vi "HandleSuffix.vi"(8 "error in (no error)":errorcluster, 11 "S4GUI in":refnum<class "S4GUI.lvclass">) -> (0 "error out":errorcluster, 3 "S4GUI out":refnum<class "S4GUI.lvclass">)   [LabVIEW 2018, in "S4GUI.lvclass"]
uses:
  S4GUI.lvclass
  S4GUI.lvclass/S4GUI.ctl
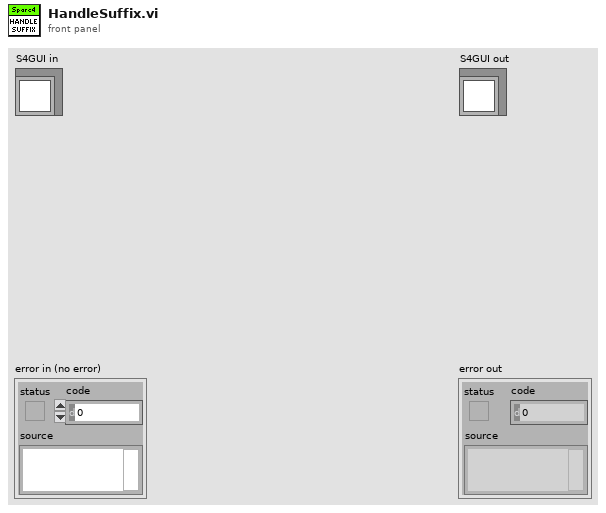
[diagram p1: front panel]
types:
  T1 = enum32{"OBJECT", "TEST", "DFLAT", "SFLAT", "DARK", "ZERO", "FOCUS"}
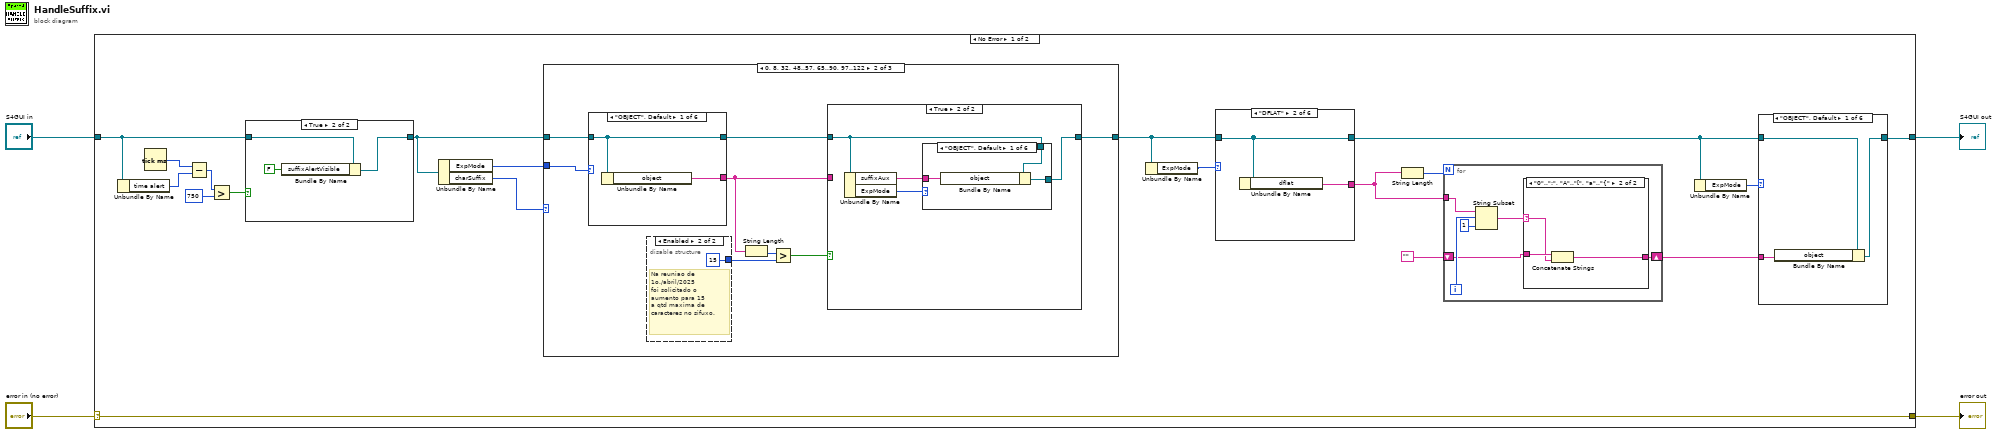
[diagram p0: block diagram]
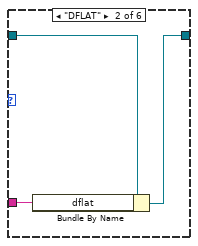
[diagram p2: hidden frame]
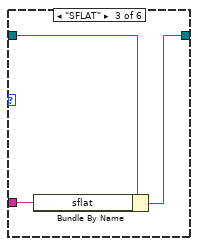
[diagram p3: hidden frame]
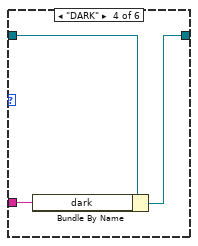
[diagram p4: hidden frame]
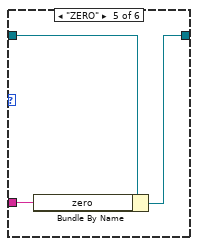
[diagram p5: hidden frame]
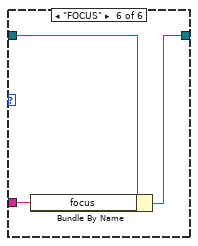
[diagram p6: hidden frame]
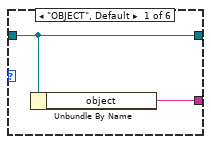
[diagram p8: hidden frame]
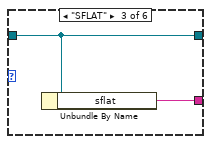
[diagram p9: hidden frame]
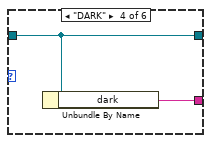
[diagram p10: hidden frame]
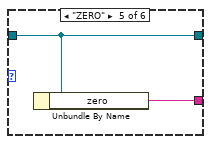
[diagram p11: hidden frame]
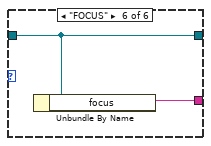
[diagram p12: hidden frame]
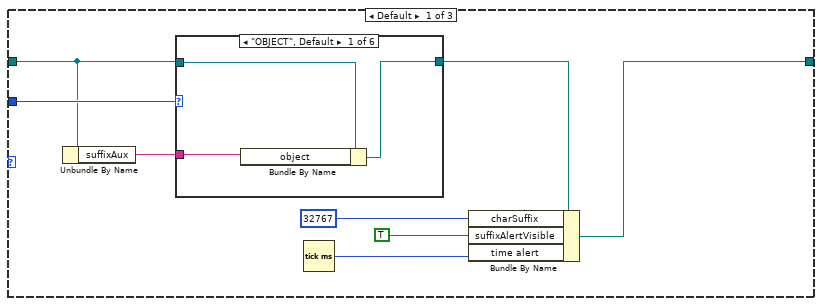
[diagram p13: hidden frame]
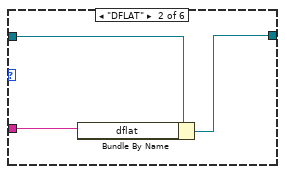
[diagram p14: hidden frame]
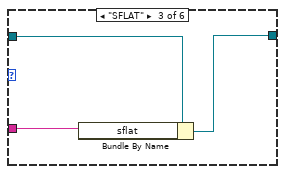
[diagram p15: hidden frame]
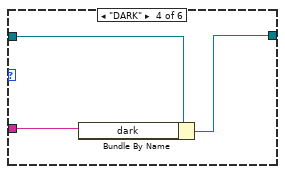
[diagram p16: hidden frame]
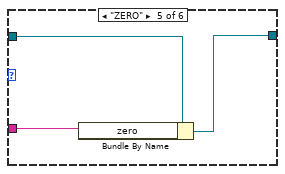
[diagram p17: hidden frame]
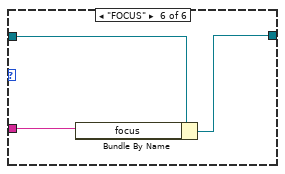
[diagram p18: hidden frame]
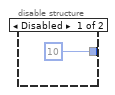
[diagram p19: hidden frame]
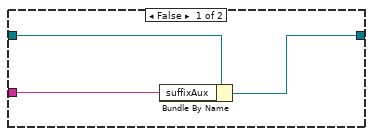
[diagram p20: hidden frame]
diagram:
  n1 = case shown="No Error" "error in (no error)" {
    selector: "error in (no error)" -> [w23 w143]
    tunnel: [w23 w143] -> w3
    tunnel: [w6 w142] -> w1
    tunnel: "S4GUI in" -> [w18 w142]
    frame No Error {
      n2 = Unbundle By Name(w18) -> ("time alert"=w20:u32)
      n3 = Tick Count (ms)() -> (millisecond timer value=w21:u32)
      n4 = Subtract(x=w21, y=w20) -> (x-y=w22:u32)
      n5 = Greater?(x=w22, y=u32 750) -> (0:w17:bool)
      n6 = case shown="True" w17 {
        tunnel: w18 -> [w138 w141]
        tunnel: [w138 w140] -> w15
        frame False {
        }
        frame True {
          n7 = Bundle By Name(cluster=w141, "suffixAlertVisible"=FALSE) -> (w140:refnum<class "S4GUI.lvclass">)
        }
      }
      n8 = Unbundle By Name(w15) -> ("ExpMode"=w16:T1, "charSuffix"=w14:i16)
      n9 = case shown="0, 8, 32, 48..57, 65..90, 97..122" w14 {
        tunnel: w15 -> [w70 w97 w137]
        tunnel: w16 -> [w71 w96 _]
        tunnel: [w64 w91 w137] -> w12
        frame Default {
          n10 = Unbundle By Name(w70) -> ("suffixAux"=w69:string)
          n11 = case shown="\"OBJECT\", Default" w71 {
            tunnel: w70 -> [w74 w77 w80 w83 w86 w89]
            tunnel: [w73 w76 w79 w82 w85 w88] -> w68
            tunnel: w69 -> [w72 w75 w78 w81 w84 w87]
            frame "OBJECT", Default {
              n12 = Bundle By Name(cluster=w74, "object"=w72) -> (w73:refnum<class "S4GUI.lvclass">)
            }
            frame "DFLAT" {
              n13 = Bundle By Name(cluster=w77, "dflat"=w75) -> (w76:refnum<class "S4GUI.lvclass">)
            }
            frame "SFLAT" {
              n14 = Bundle By Name(cluster=w80, "sflat"=w78) -> (w79:refnum<class "S4GUI.lvclass">)
            }
            frame "DARK" {
              n15 = Bundle By Name(cluster=w83, "dark"=w81) -> (w82:refnum<class "S4GUI.lvclass">)
            }
            frame "ZERO" {
              n16 = Bundle By Name(cluster=w86, "zero"=w84) -> (w85:refnum<class "S4GUI.lvclass">)
            }
            frame "FOCUS" {
              n17 = Bundle By Name(cluster=w89, "focus"=w87) -> (w88:refnum<class "S4GUI.lvclass">)
            }
          }
          n18 = Tick Count (ms)() -> (millisecond timer value=w65:u32)
          n19 = Bundle By Name(cluster=w68, "charSuffix"=i16 32767, "suffixAlertVisible"=TRUE, "time alert"=w65) -> (w64:refnum<class "S4GUI.lvclass">)
        }
        frame 0, 8, 32, 48..57, 65..90, 97..122 {
          n20 = case shown="\"OBJECT\", Default" w96 {
            tunnel: w97 -> [w126 w128 w130 w132 w134 w136]
            tunnel: [w126 w128 w130 w132 w134 w136] -> w92
            tunnel: [w125 w127 w129 w131 w133 w135] -> w90
            frame "OBJECT", Default {
              n21 = Unbundle By Name(w126) -> ("object"=w125:string)
            }
            frame "DFLAT" {
              n22 = Unbundle By Name(w128) -> ("dflat"=w127:string)
            }
            frame "SFLAT" {
              n23 = Unbundle By Name(w130) -> ("sflat"=w129:string)
            }
            frame "DARK" {
              n24 = Unbundle By Name(w132) -> ("dark"=w131:string)
            }
            frame "ZERO" {
              n25 = Unbundle By Name(w134) -> ("zero"=w133:string)
            }
            frame "FOCUS" {
              n26 = Unbundle By Name(w136) -> ("focus"=w135:string)
            }
          }
          n27 = disable-structure shown="Enabled" {
            disable-tunnel: [10 ("y") 15 ("y")] -> w94
            frame Disabled {
            }
            frame Enabled {
              # "Na reuniao de \n1o./abril/2025\nfoi solicitado o \naumento para 15\na qtd maxima de\ncaracteres no sifuxo."
            }
          }
          n28 = String Length(string=w90) -> (length=w95:i32)
          n29 = Greater?(x=w95, y=w94) -> (0:w93:bool)
          n30 = case shown="True" w93 {
            tunnel: w92 -> [w102 w106]
            tunnel: [w101 w105] -> w91
            tunnel: w90 -> [w100 _]
            frame False {
              n31 = Bundle By Name(cluster=w102, "suffixAux"=w100) -> (w101:refnum<class "S4GUI.lvclass">)
            }
            frame True {
              n32 = Unbundle By Name(w106) -> ("suffixAux"=w103:string, "ExpMode"=w104:T1)
              n33 = case shown="\"OBJECT\", Default" w104 {
                tunnel: w106 -> [w109 w112 w115 w118 w121 w123]
                tunnel: [w108 w111 w114 w117 w120 w122] -> w105
                tunnel: w103 -> [w107 w110 w113 w116 w119 w124]
                frame "OBJECT", Default {
                  n34 = Bundle By Name(cluster=w109, "object"=w107) -> (w108:refnum<class "S4GUI.lvclass">)
                }
                frame "DFLAT" {
                  n35 = Bundle By Name(cluster=w112, "dflat"=w110) -> (w111:refnum<class "S4GUI.lvclass">)
                }
                frame "SFLAT" {
                  n36 = Bundle By Name(cluster=w115, "sflat"=w113) -> (w114:refnum<class "S4GUI.lvclass">)
                }
                frame "DARK" {
                  n37 = Bundle By Name(cluster=w118, "dark"=w116) -> (w117:refnum<class "S4GUI.lvclass">)
                }
                frame "ZERO" {
                  n38 = Bundle By Name(cluster=w121, "zero"=w119) -> (w120:refnum<class "S4GUI.lvclass">)
                }
                frame "FOCUS" {
                  n39 = Bundle By Name(cluster=w123, "focus"=w124) -> (w122:refnum<class "S4GUI.lvclass">)
                }
              }
            }
          }
        }
        frame 32767 {
        }
      }
      n40 = Unbundle By Name(w12) -> ("ExpMode"=w13:T1)
      n41 = case shown="\"DFLAT\"" w13 {
        tunnel: w12 -> [w53 w55 w57 w59 w61 w63]
        tunnel: [w52 w54 w56 w58 w60 w62] -> w10
        tunnel: [w53 w55 w57 w59 w61 w63] -> w7
        frame "OBJECT", Default {
          n42 = Unbundle By Name(w53) -> ("object"=w52:string)
        }
        frame "DFLAT" {
          n43 = Unbundle By Name(w55) -> ("dflat"=w54:string)
        }
        frame "SFLAT" {
          n44 = Unbundle By Name(w57) -> ("sflat"=w56:string)
        }
        frame "DARK" {
          n45 = Unbundle By Name(w59) -> ("dark"=w58:string)
        }
        frame "ZERO" {
          n46 = Unbundle By Name(w61) -> ("zero"=w60:string)
        }
        frame "FOCUS" {
          n47 = Unbundle By Name(w63) -> ("focus"=w62:string)
        }
      }
      n48 = String Length(string=w10) -> (length=w11:i32)
      n49 = for {
        N: w11 -> [_]
        tunnel: w10 -> [w47]
        shift-right: [w42] -> w5
        shift-left: "" -> [w44]
        i -> [w46]
        n50 = String Subset(string=w47, offset (0)=w46, length (rest)=1 ("length (rest)")) -> (substring=w43:string)
        n51 = case shown="\"0\"..\":\", \"A\"..\"[\", \"a\"..\"{\"" w43 {
          selector: w43 -> [_ w50]
          tunnel: w44 -> [w48 w51]
          tunnel: [w48 w49] -> w42
          frame Default {
          }
          frame "0"..":", "A".."[", "a".."{" {
            n52 = Concatenate Strings(w51, w50) -> (w49:string)
          }
        }
      }
      n53 = Unbundle By Name(w7) -> ("ExpMode"=w8:T1)
      n54 = case shown="\"OBJECT\", Default" w8 {
        tunnel: w7 -> [w26 w29 w32 w35 w38 w41]
        tunnel: [w25 w28 w31 w34 w37 w40] -> w6
        tunnel: w5 -> [w24 w27 w30 w33 w36 w39]
        frame "OBJECT", Default {
          n55 = Bundle By Name(cluster=w26, "object"=w24) -> (w25:refnum<class "S4GUI.lvclass">)
        }
        frame "DFLAT" {
          n56 = Bundle By Name(cluster=w29, "dflat"=w27) -> (w28:refnum<class "S4GUI.lvclass">)
        }
        frame "SFLAT" {
          n57 = Bundle By Name(cluster=w32, "sflat"=w30) -> (w31:refnum<class "S4GUI.lvclass">)
        }
        frame "DARK" {
          n58 = Bundle By Name(cluster=w35, "dark"=w33) -> (w34:refnum<class "S4GUI.lvclass">)
        }
        frame "ZERO" {
          n59 = Bundle By Name(cluster=w38, "zero"=w36) -> (w37:refnum<class "S4GUI.lvclass">)
        }
        frame "FOCUS" {
          n60 = Bundle By Name(cluster=w41, "focus"=w39) -> (w40:refnum<class "S4GUI.lvclass">)
        }
      }
    }
    frame Error {
    }
  }
  "error out" <- w3
  "S4GUI out" <- w1
